vi "Start Device.vi"(8 "error in":errorcluster, 11 "DAQ Device in":refnum<class "DAQ Device.lvclass">) -> (0 "error out":errorcluster, 3 "DAQ Device out":refnum<class "DAQ Device.lvclass">)   [LabVIEW 2014, in "DAQ Device.lvclass"]
uses:
  DAQ Device.lvclass
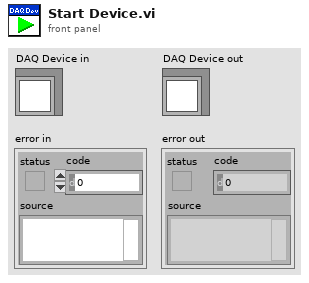
[diagram p1: front panel]
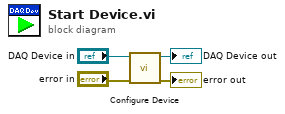
[diagram p0: block diagram]
diagram:
  n1 = call-dynamic "Configure Device.vi"("error in"="error in", "DAQ Device in"="DAQ Device in") -> ("error out"=→"error out":errorcluster, "DAQ Device out"=→"DAQ Device out":refnum<class "DAQ Device.lvclass">)  [unwired: 8 in]
